vi "Remove Guardian.vi"(8 "error in (no error)":errorcluster, 10 "Guardian ID":string, 11 "Distr uS Map ref in":refnum<data-value>) -> (0 "error out":errorcluster, 3 "Distr uS Map ref out":refnum<data-value>)   [LabVIEW 2026, in "TALOS.lvlib" / "Classes.lvlib" / "Distributed uService Map.lvclass"]
uses:
  Distributed uService Map.lvclass
  Distributed uService Map.lvclass/Distributed uService Map.ctl
  Ancestor/Ancestor/Ancestor.lvclass/Ancestor.ctl
  93f74587-5752-48d2-aff7-fa68ae622b14.vi
  Support VIs/Generate Error.vi
  FGV/Error Memory/Get Error Description.vi
  Support VIs/Get PC name.vi
  Ancestor/Ancestor/Read ID.vi
  Support VIs/Get Class Name.vi
  <vilib>/Utility/error.llb/Clear Errors.vi
  FGV/Error Memory/Error Memory Core.vi
  <vilib>/AdvancedString/Delimited String to 1D String Array.vi
  <vilib>/AdvancedString/Delimited String to 1D String Array (string).vi
  Support VIs/Circus Root Path.vi
  FGV/Error Memory/Error Crt Lvl checker.vi
  FGV/Error Memory/Error Memory Core.vi/40c8088d-b597-4017-91af-faa98e00292e.vi
  FGV/Error Memory/Error Memory Core.vi/d4a3ab98-063c-4e44-b43d-fbdcfe6c2be2.vi
  Support VIs/Global Memory.vi
  <vilib>/Utility/LVClass/Get LV Class Name.vi
  Support VIs/Is in Packed Library.vi
  Support VIs/TALOS Root path.vi
  Support VIs/Read CSV worksheet.vi
  Support VIs/Global Constants.vi
  <vilib>/Utility/error.llb/General Error Handler.vi
  Support VIs/Error Log.vi
  <vilib>/Comparison/Equal/Equal Functor/Equal Functor.lvclass
  Ancestor/Ancestor/Ancestor.lvclass
  TALOS.lvlib
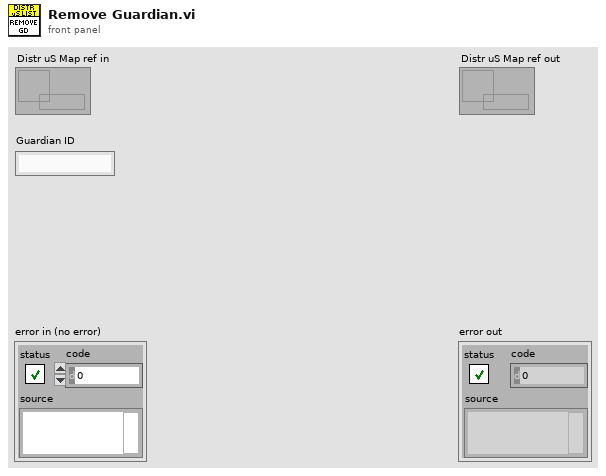
[diagram p1: front panel]
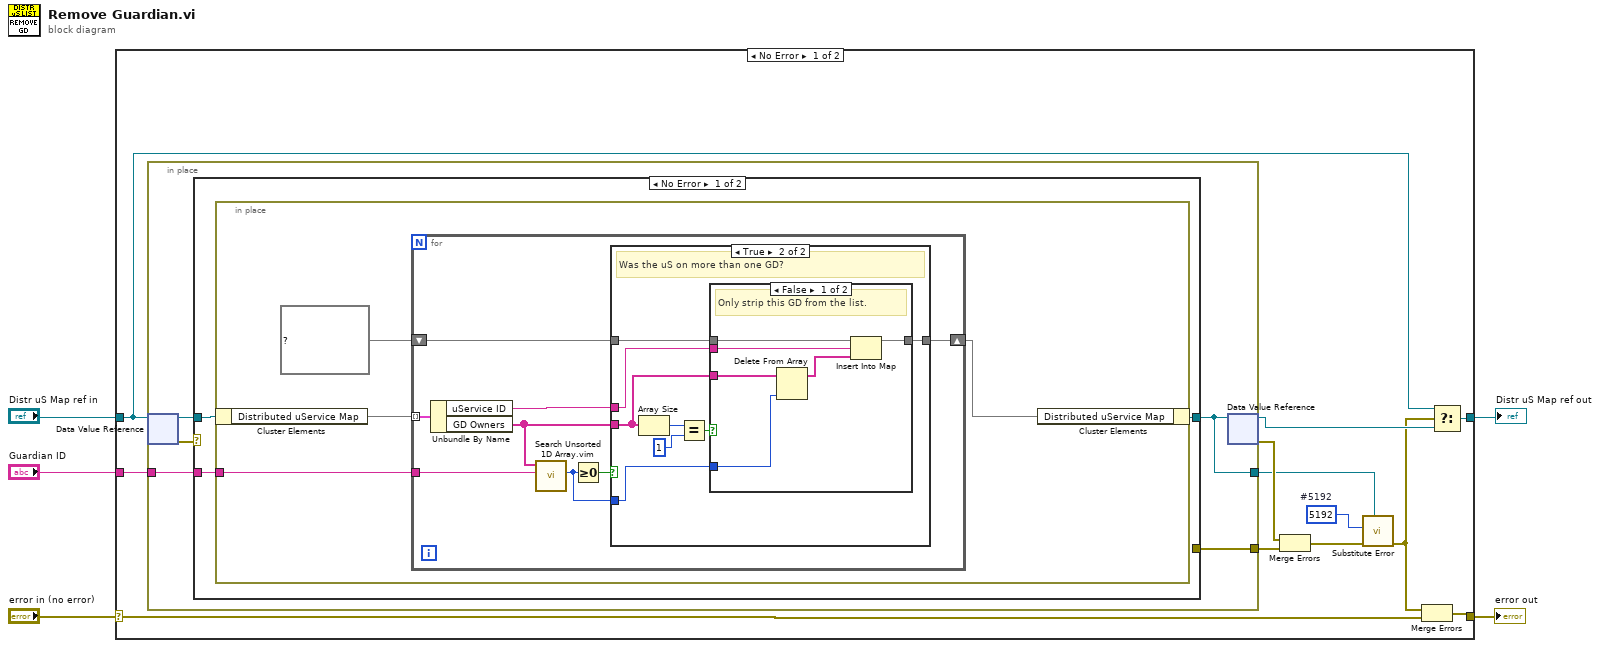
[diagram p0: block diagram]
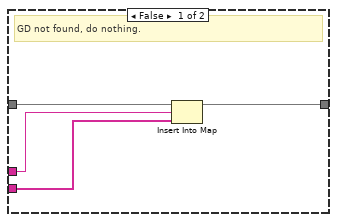
[diagram p2: hidden frame]
diagram:
  n1 = case shown="No Error" "error in (no error)" {
    selector: "error in (no error)" -> [w12 w60]
    tunnel: [w11 w60] -> w4
    tunnel: [w16 w59] -> w2
    tunnel: "Distr uS Map ref in" -> [w15 w59]
    tunnel: "Guardian ID" -> [w17 _]
    frame No Error {
      w6 = 5192  # #5192
      n2 = in-place {
        in-place-border: w17 -> [w22]
        in-place-border: [w19] -> w14
        in-place-border: [w18] -> w9
        n3 = in-place-dvr #1(w15) -> (w21:refnum<class "Distributed uService Map.lvclass">, w20:errorcluster)
        n4 = case shown="No Error" w20 {
          selector: w20 -> [_ w57]
          tunnel: [w25 w58] -> w18
          tunnel: w22 -> [w24 _]
          tunnel: w21 -> [w23 w58]
          tunnel: [_ w57] -> w19
          frame No Error {
            n5 = in-place {
              in-place-border: w24 -> [w28]
              n6 = in-place-cluster #2(w23) -> ("Distributed uService Map"=w29:map{string, string[]})
              n7 = for {
                tunnel: w29 -> [w37] mode=indexing
                tunnel: w28 -> [w36]
                shift-right: [w31] -> w26
                shift-left: map{string, string[]} {} ("Distributed uService Map") -> [w32]
                n8 = Unbundle By Name(w37) -> ("uService ID"=w34:string, "GD Owners"=w33:string[])
                n9 = call "Search Unsorted 1D Array.vim"("element"=w36, "unsorted 1D array"=w33) -> ("index of element"=w30:i32)  [unwired: 9 in]
                n10 = Greater Or Equal To 0?(x=w30) -> (x >= 0?=w35:bool)
                n11 = case shown="True" w35 {
                  tunnel: w34 -> [w40 w43]
                  tunnel: w33 -> [w39 w42]
                  tunnel: w32 -> [w41 w46]
                  tunnel: [w38 w45] -> w31
                  tunnel: w30 -> [_ w44]
                  frame False {
                    # "GD not found, do nothing."
                    n12 = Insert Into Map(map in=w41, key=w40, value=w39) -> (map out=w38:map{string, string[]})  [unwired: 2 out]
                  }
                  frame True {
                    # "Was the uS on more than one GD?"
                    n13 = Array Size(array=w42) -> (size(s)=w49:i32)
                    n14 = Equal?(x=w49, y=1) -> (x = y?=w47:bool)
                    n15 = case shown="False" w47 {
                      tunnel: w46 -> [w55 w56]
                      tunnel: [w54 w56] -> w45
                      tunnel: w44 -> [w50 _]
                      tunnel: w43 -> [w53 _]
                      tunnel: w42 -> [w52 _]
                      frame False {
                        # "Only strip this GD from the list."
                        n16 = Delete From Array(array=w52, index=w50) -> (array with subset deleted=w51:string[])  [unwired: 1 in, 1 out]
                        n17 = Insert Into Map(map in=w55, key=w53, value=w51) -> (map out=w54:map{string, string[]})  [unwired: 2 out]
                      }
                      frame True {
                        # "It was the only GD with this uS: remove it from the list."
                      }
                    }
                  }
                }
              }
              n18 = in-place-cluster #2("Distributed uService Map"=w26) -> (w25:refnum<class "Distributed uService Map.lvclass">)
            }
          }
          frame Error {
          }
        }
        n19 = in-place-dvr #1(w18) -> (w8:refnum<data-value>, w13:errorcluster)
      }
      n20 = Merge Errors(w13, w14) -> (w10:errorcluster)
      n21 = call "Substitute Error.vi"("LabVIEW Object"=w9, "error in (no error)"=w10, "Error Code"=w6) -> ("error out"=w7:errorcluster)  [unwired: 8 in]
      n22 = Merge Errors(w7, w12) -> (w11:errorcluster)
      n23 = Select(t=w15, s=w7, f=w8) -> (s? t:f=w16:refnum<data-value>)
    }
    frame Error {
    }
  }
  "error out" <- w4
  "Distr uS Map ref out" <- w2
